vi "Acquire Data.vi"() -> (0 "Time Waveform":waveform(dbl)(graph))   [LabVIEW 2010]
doc: "This VI either acquires data from a data acquisition (DAQ) board or generates a noisy sine waveform. Then the frequency response is calculated and displayed with the time waveform in waveform graphs. Correct error handling is emphasized using the error clusters and the Simple Error Handler VI."
uses:
  <vilib>/measure/maspectr.llb/FFT Power Spectrum for 1 Chan.vi
  <vilib>/measure/NI_MABase.lvlib
  <vilib>/measure/NI_MAPro.lvlib
panel:
  in  "Tab Control":enum32{"Simulate"}(tab)
  in  "Sampling Info":cluster{"Fs":dbl, "#s":dbl}={"Fs"=1000.0, "#s"=500.0} {"#s" format="%0.2p"; "Fs" format="%0.2p"}
  in  "Noise Amplitude":dbl(slide)=1.0 scale=0.0..10.0
  in  "Sine Amplitude":dbl(slide)=1.0 scale=0.0..10.0
  in  "Sine Frequency":dbl(slide)=100.0 scale=0.0..500.0 scale format="%0.1f"
  in  "Averaging Parameters":T1={"averaging mode"=enum."No averaging", "weighting mode"=enum."Exponential", "number of averages"=10} {"number of averages" min=1}
  in  "stop":bool
  out "Power Spectrum":cluster{"f0":dbl, "df":dbl, "magnitude":dbl[]}(graph)
  # "Change the data by adjusting the parameters on the Simulate tab.  The choices listed under Averaging\nParameters can be varied to change the treatment of the data.  Press the Continue button when finished."
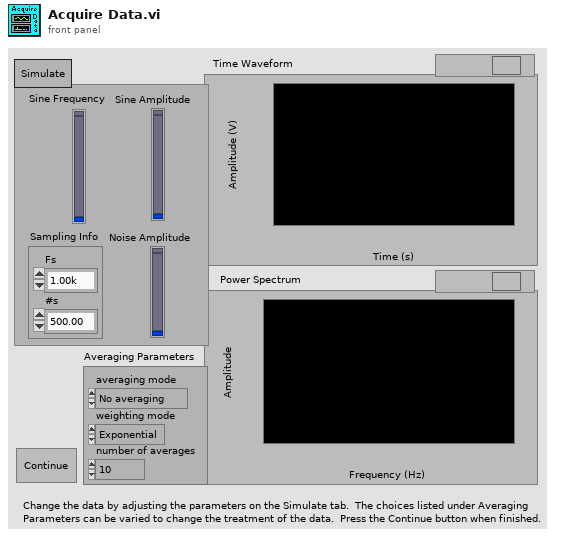
[diagram p1: front panel]
types:
  T1 = cluster{"averaging mode":enum16{"No averaging", "Vector averaging", "RMS averaging", "Peak hold"}, "weighting mode":enum16{"Linear", "Exponential"}, "number of averages":u32}
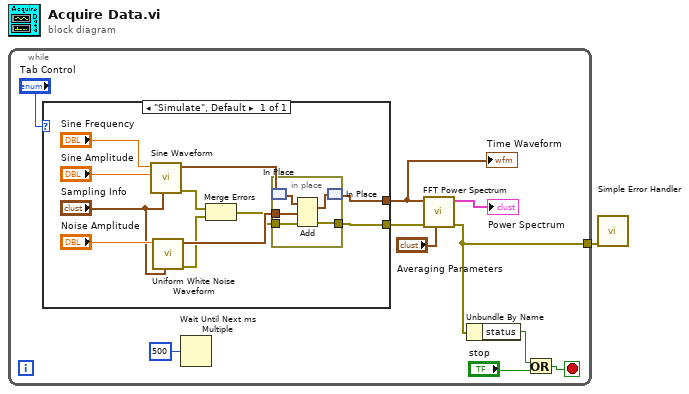
[diagram p0: block diagram]
diagram:
  n1 = while {
    tunnel: [w4] -> w1
    stop <- w5 stop-if-true
    n2 = case shown="\"Simulate\", Default" "Tab Control" {
      tunnel: [w15] -> w11
      tunnel: [w12] -> w3
      frame "Simulate", Default {
        n3 = call <vilib>:"Sine Waveform.vi"("sampling info"="Sampling Info", "amplitude"="Sine Amplitude", "frequency"="Sine Frequency") -> ("error out"=w17:errorcluster, "signal out"=w20:waveform(dbl))  [unwired: 7 in]
        n4 = call <vilib>:"Uniform White Noise Waveform.vi"("sampling info"="Sampling Info", "amplitude"="Noise Amplitude") -> ("error out"=w18:errorcluster, "signal out"=w19:waveform(dbl))  [unwired: 8 in]
        n5 = Merge Errors(w17, w18) -> (w16:errorcluster)
        n6 = in-place {
          in-place-border: w19 -> [w26]
          in-place-border: w16 -> [w25]
          in-place-border: [w24] -> w15
          n7 = in-place-match #1(w20) -> (w27:waveform(dbl))
          n8 = Add(1:w26, 2:w27, 4:w25) -> (0:w23:waveform(dbl), 3:w24:errorcluster)
          n9 = in-place-match #1(w23) -> (w12:waveform(dbl))
        }
      }
    }
    "Time Waveform" <- w3
    n10 = Wait Until Next ms Multiple(millisecond multiple=u32 500) -> ()  [unwired: 1 out]
    n11 = call-poly <vilib>:"FFT Power Spectrum.vi"("averaging parameters"="Averaging Parameters", "error in (no error)"=w11, "time signal"=w3) -> ("error out"=w4:errorcluster, "power spectrum"=→"Power Spectrum":cluster{"f0":dbl, "df":dbl, "magnitude":dbl[]})  [unwired: 5 in, 2 out]
    n12 = Unbundle By Name "Unbundle By Name"(w4) -> ("status"=w7:bool)
    n13 = Or(x=w7, y="stop") -> (x .or. y?=w5:bool)
  }
  n14 = call <vilib>:"Simple Error Handler.vi"("error in (no error)"=w1) -> ()  [unwired: 4 in, 5 out]
